vi "USB config low.vi"(0 "Port":refnum<visa-resource-name>, 1 "Tx msg cluster":T1={"addr"=1, "cmd"="A", "data (float)"=0.0}, 2 "Error in":errorcluster) -> (3 "Port out":refnum<visa-resource-name>, 4 "Value returned":sgl, 6 "Error out":errorcluster)   [LabVIEW 2017]
uses:
  ctls/USB Tx msg cluster.ctl
panel:
  out "Bytes returned":u32
  out "Read buffer (hex)":string
  out "Write buffer (hex)":string
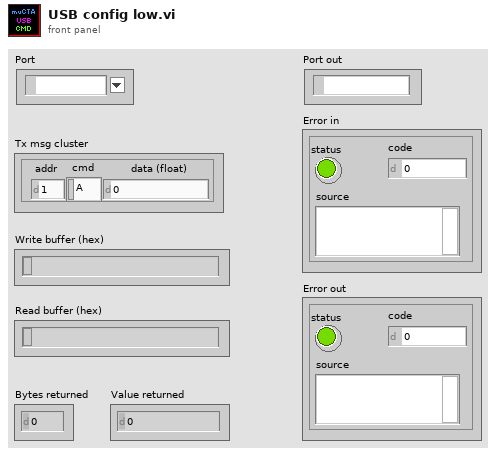
[diagram p1: front panel]
types:
  T1 = typedef "USB Tx msg cluster.ctl" = cluster{"addr":u8, "cmd":string, "data (float)":sgl}
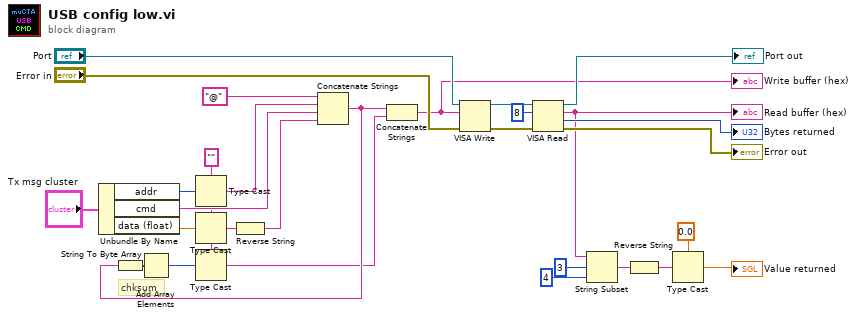
[diagram p0: block diagram]
diagram:
  w5 = ""
  # "chksum"
  n1 = Unbundle By Name("Tx msg cluster") -> ("addr"=w23:u8, "cmd"=w10:string, "data (float)"=w22:sgl)
  n2 = Type Cast(type=w5, x=w23) -> (*(type *) &x=w11:string)
  n3 = Type Cast(type=w5, x=w22) -> (*(type *) &x=w9:string)
  n4 = Reverse String(1:w9) -> (0:w2:string)
  n5 = Concatenate Strings("@", w11, w10, w2) -> (w7:string)
  n6 = String To Byte Array(string=w7) -> (unsigned byte array=w6:u8[])
  n7 = Add Array Elements(numeric array=w6) -> (sum=w4:u8)
  n8 = Type Cast(type=w5, x=w4) -> (*(type *) &x=w3:string)
  n9 = Concatenate Strings(w7, w3) -> (w8:string)
  "Write buffer (hex)" <- w8
  n10 = VISA Write(VISA resource name="Port", write buffer=w8, error in (no error)="Error in") -> (VISA resource name out=w25:refnum<visa-resource-name>, error out=w28:errorcluster)  [unwired: 1 out]
  n11 = VISA Read(VISA resource name=w25, byte count=u32 8, error in (no error)=w28) -> (VISA resource name out=→"Port out":refnum<visa-resource-name>, read buffer=w14:string, return count=→"Bytes returned":u32, error out=→"Error out":errorcluster)
  "Read buffer (hex)" <- w14
  n12 = String Subset(string=w14, offset (0)=3, length (rest)=4 ("length (rest)")) -> (substring=w19:string)
  n13 = Reverse String(1:w19) -> (0:w1:string)
  n14 = Type Cast(type=sgl 0.0, x=w1) -> (*(type *) &x=→"Value returned":sgl)
